vi "LabVIEW to JSON.vi"(8 "error in (no error)":errorcluster, 10 "Data":dbl) -> (0 "error out":errorcluster, 3 "JSON out":refnum<class "JSON Datatype.lvclass">)   [LabVIEW 2015, in "LVJSON.lvlib" / "JSON Datatype.lvclass"]
uses:
  JSON Datatype.lvclass
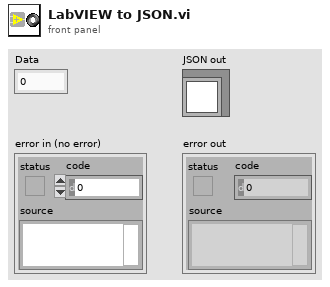
[diagram p1: front panel]
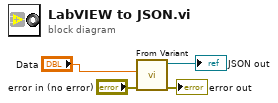
[diagram p0: block diagram]
diagram:
  n1 = call "From Variant.vi"("error in (no error)"="error in (no error)", "Variant"="Data") -> ("error out"=→"error out":errorcluster, "JSON out"=→"JSON out":refnum<class "JSON Datatype.lvclass">)  [unwired: 8 in]
